vi "DDPoseEst2_AbsTraj_Work.vi"(5 "Track Width FT":dbl, 7 "Max Speed\nFT/SEC":dbl, 8 "Init":bool) -> (0 "AtReference":bool, 1 "Right Speed Target":dbl, 2 "Left Speed Target":dbl, 4 "Odometry Pose Meters":T1={"TRANSLATION"={"X"=0.0, "Y"=0.0}, "ROTATION"={"VALUE"=0.0, "COS"=1.0, "SIN"=0.0}} {"ROTATION"."SIN" format="%13.4f"; "ROTATION"."COS" format="%13.4f"; "ROTATION"."VALUE" format="%13.4f"; "TRANSLATION"."Y" format="%14.3f"; "TRANSLATION"."X" format="%14.3f"})   [LabVIEW 2019]
uses:
  <vilib>/Rock Robotics/WPI/ThirdParty/JAS_Junk/TrajLib/Trajectory_Library.lvlib
  DDPoseEst2_Traj_Globals.vi
  <vilib>/Rock Robotics/WPI/ThirdParty/JAS_Junk/TrajLib/TypeDef/TRANSLATION2D.ctl
  <vilib>/Rock Robotics/WPI/ThirdParty/JAS_Junk/TrajLib/TypeDef/ROTATION2D.ctl
  <vilib>/Rock Robotics/WPI/ThirdParty/JAS_Junk/TrajLib/TypeDef/POSE2D.ctl
  <vilib>/Rock Robotics/WPI/ThirdParty/JAS_Junk/TrajLib/TypeDef/TRAJ_STATE.ctl
  <vilib>/Rock Robotics/WPI/ThirdParty/JAS_Junk/TrajLib/TypeDef/TRAJECTORY.ctl
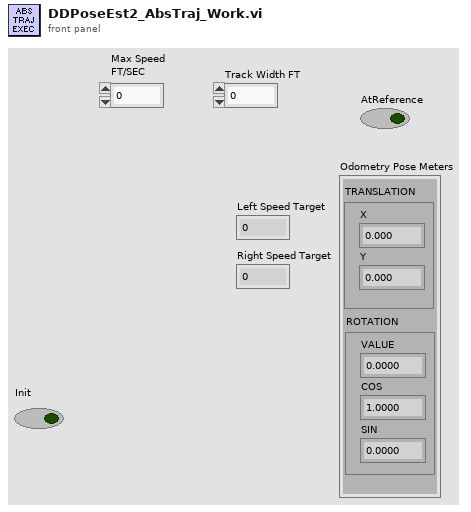
[diagram p1: front panel]
types:
  T1 = typedef "Trajectory_Library.lvlib/POSE2D.ctl" = cluster{"TRANSLATION":T2, "ROTATION":T3}
  T2 = typedef "Trajectory_Library.lvlib/TRANSLATION2D.ctl" = cluster{"X":dbl, "Y":dbl}
  T3 = typedef "Trajectory_Library.lvlib/ROTATION2D.ctl" = cluster{"VALUE":dbl, "COS":dbl, "SIN":dbl}
  T4 = typedef "Trajectory_Library.lvlib/TRAJECTORY.ctl" = cluster{"TotalTImeSecs":dbl, "States":T5[]}
  T5 = typedef "Trajectory_Library.lvlib/TRAJ_STATE.ctl" = cluster{"TimeSeconds":dbl, "Velocity":dbl, "Acceleration":dbl, "POSE":T1, "Curvature":dbl}
  T6 = typedef "Trajectory_Library.lvlib/WEIGHTED_WAYPOINT.ctl" = cluster{"TRANSLATION":T2, "ROTATION":T3, "SCALAR":dbl}
  T7 = typedef "Trajectory_Library.lvlib/RAMSETE_EXE_TUNING.ctl" = cluster{"B":dbl, "Zeta":dbl, "X Tolerance M":dbl, "Y Tolerance M":dbl, "Heading Tolerance RAD":dbl, "Track Width M":dbl, "Max Speed M/S":dbl}
  T8 = typedef "Trajectory_Library.lvlib/RAMSETE.ctl" = cluster{"B":dbl, "Zeta":dbl, "poseTolerance":T1, "poseError":T1, "Enabled":bool}
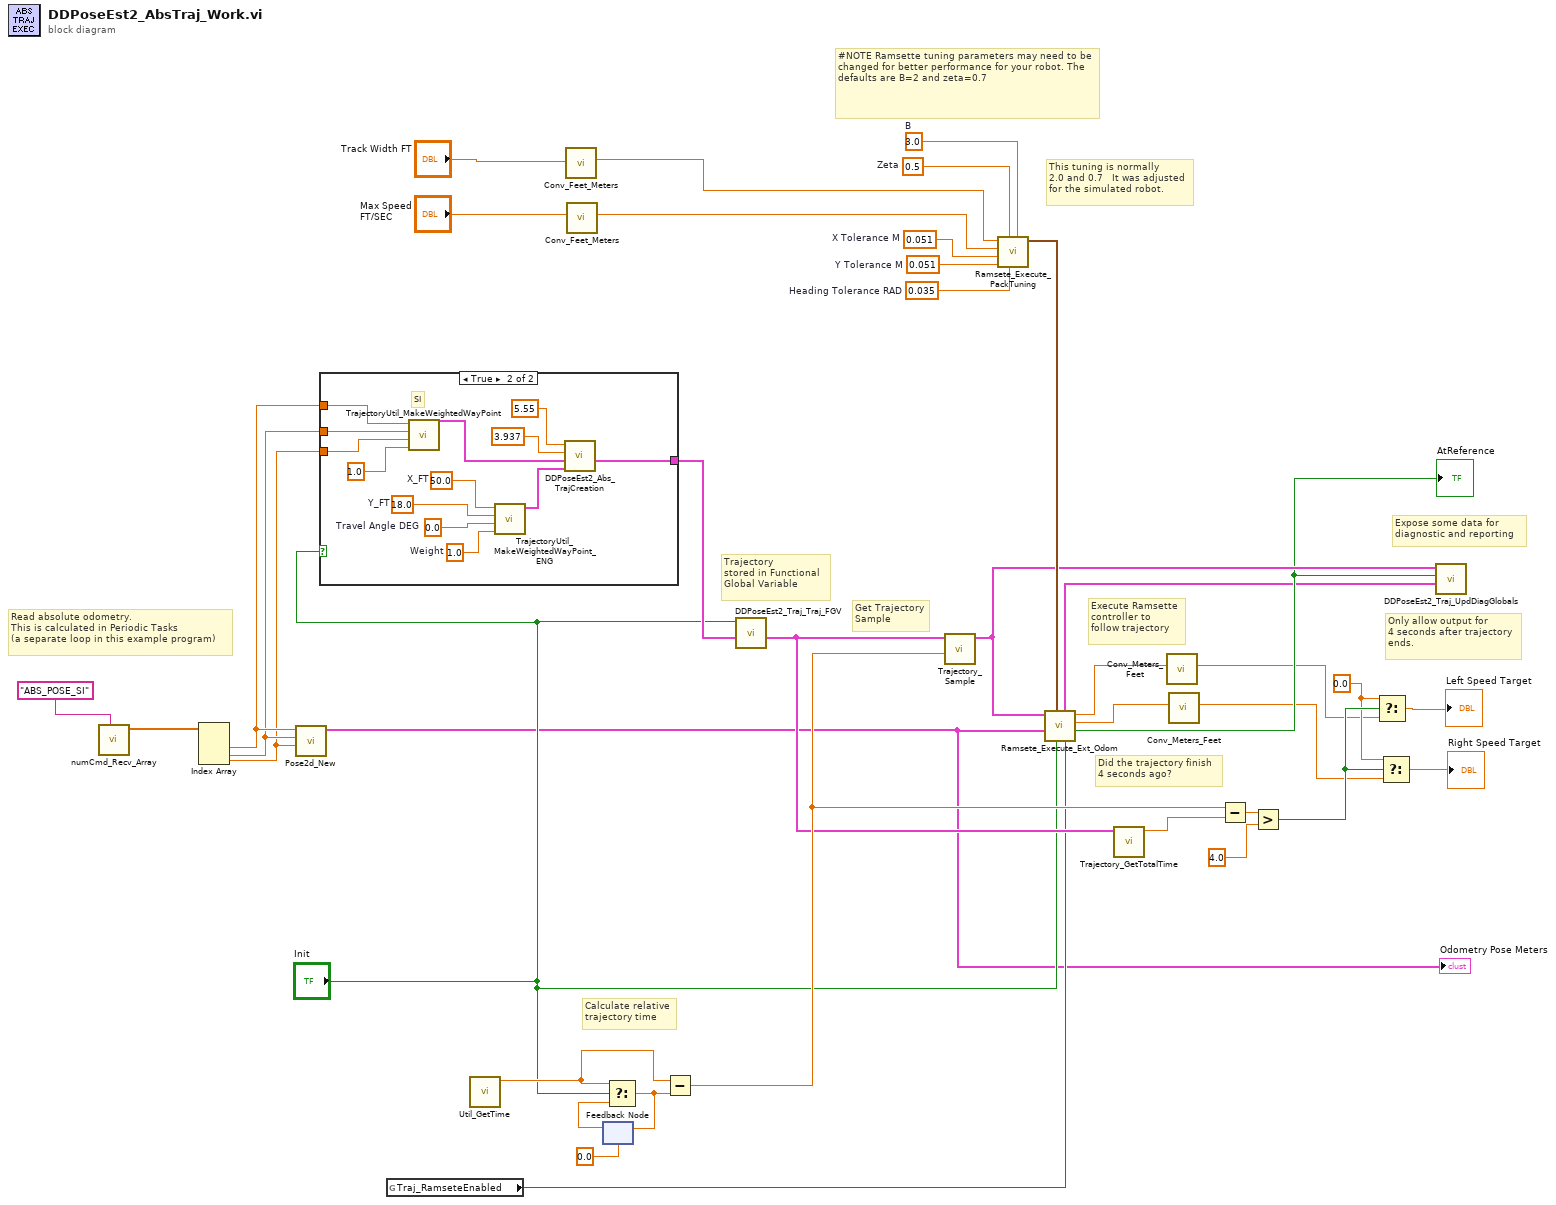
[diagram p0: block diagram]
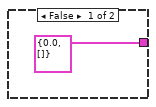
[diagram p2: hidden frame]
diagram:
  w27 = 0.051  # X Tolerance M
  w26 = 0.051  # Y Tolerance M
  w25 = 0.5  # Zeta
  w24 = 0.035  # Heading Tolerance RAD
  w23 = 3.0  # B
  w34 = 0.0 ("t")
  # "Read absolute odometry. \nThis is calculated in Periodic Tasks\n(a separate loop in this example program)"
  # "Execute Ramsette\ncontroller to \nfollow trajectory"
  # "This tuning is normally\n2.0 and 0.7   It was adjusted\nfor the simulated robot."
  # "Expose some data for\ndiagnostic and reporting"
  # "Did the trajectory finish\n4 seconds ago?"
  # "Get Trajectory\nSample"
  # "Trajectory\nstored in Functional\nGlobal Variable"
  # "Calculate relative\ntrajectory time"
  # "#NOTE Ramsette tuning parameters may need to be changed for better performance for your robot. The defaults are B=2 and zeta=0.7"
  # "Only allow output for\n4 seconds after trajectory\nends."
  n1 = call <vilib>:"numCmd_Recv_Array.vi"("Command Name"="ABS_POSE_SI") -> ("Values"=w7:dbl[])  [unwired: 8 in, 2 out]
  n2 = Index Array(array=w7) -> (element #1=w3:dbl, element #2=w2:dbl, element #3=w1:dbl)  [unwired: 3 in]
  n3 = call <vilib>:"Pose2d_New.vi"("Heading"=w1, "Y"=w2, "X"=w3) -> ("out POSe"=w4:T1)  [unwired: 8 in]
  "Odometry Pose Meters" <- w4
  n4 = case shown="True" "Init" {
    tunnel: [T4 {"TotalTImeSecs"=0.0, "States"=[]} ("Absolute Trajectory") w53] -> w6
    tunnel: w3 -> [_ w50]
    tunnel: w2 -> [_ w49]
    tunnel: w1 -> [_ w48]
    frame False {
    }
    frame True {
      w42 = 50.0  # X_FT
      w43 = 18.0  # Y_FT
      w44 = 0.0  # Travel Angle DEG
      w45 = 1.0  # Weight
      # "SI"
      n5 = call <vilib>:"TrajectoryUtil_MakeWeightedWayPoint.vi"("Weight"=1.0, "Travel Angle Radians"=w48, "Y_M"=w49, "X_M"=w50) -> ("WEIGHTED_WAYPOINT"=w46:T6)  [unwired: 7 in]
      n6 = call <vilib>:"TrajectoryUtil_MakeWeightedWayPoint_ENG.vi"("Weight"=w45, "Travel Angle DEG"=w44, "Y_FT"=w43, "X_FT"=w42) -> ("WEIGHTED_WAYPOINT"=w41:T6)  [unwired: 7 in]
      n7 = call "DDPoseEst2_Abs_TrajCreation.vi"("Destination Waypoint"=w41, "Initial Waypoint"=w46, "Effective Track Width Ft"=3.937, "Max Velocity Ft/Sec"=5.55) -> ("Absolute Trajectory"=w53:T4)  [unwired: 4 in, 3 out]
    }
  }
  n8 = global read "DDPoseEst2_Traj_Globals.vi" "Traj_RamseteEnabled"() -> (w18:bool)
  n9 = call <vilib>:"Util_GetTime.vi"() -> ("FPGA_Time_Seconds"=w9:dbl)  [unwired: 9 in, 2 out]
  n10 = call <vilib>:"Conv_Feet_Meters.vi"("Feet"="Track Width FT") -> ("Meters"=w10:dbl)  [unwired: 10 in]
  n11 = call <vilib>:"Conv_Feet_Meters.vi"("Feet"="Max Speed\nFT/SEC") -> ("Meters"=w21:dbl)  [unwired: 10 in]
  n12 = feedback #1(0.0 ("TIME")) -> (w30:dbl)
  n13 = Select(t=w9, s="Init", f=w30) -> (s? t:f=w31:dbl)
  n14 = feedback-in #1(w31) -> ()
  n15 = Subtract(x=w9, y=w31) -> (x-y=w38:dbl)
  n16 = call "DDPoseEst2_Traj_Traj_FGV.vi"("inTRAJECTORY"=w6, "WRITE"="Init") -> ("outTRAJECTORY"=w29:T4)  [unwired: 9 in]
  n17 = call <vilib>:"Trajectory_Sample.vi"("Time"=w38, "InputTRAJECTORY"=w29) -> ("OutputTRAJ_STATE"=w17:T5)  [unwired: 9 in]
  n18 = call <vilib>:"Ramsete_Execute_PackTuning.vi"("B"=w23, "Heading Tolerance RAD"=w24, "Zeta"=w25, "Y Tolerance M"=w26, "X Tolerance M"=w27, "Max Speed M/S"=w21, "Track Width M"=w10) -> ("RAMSETE_EXE_TUNING"=w22:T7)  [unwired: 4 in]
  n19 = call <vilib>:"Ramsete_Execute_Ext_Odom.vi"("Enabled"=w18, "Reset"="Init", "RAMSETE_EXE_TUNING SI"=w22, "Current Pose SI"=w4, "TRAJ_STATE SI"=w17) -> ("AtReference"=w16:bool, "Right Speed Dmd M/S"=w13:dbl, "Left Speed Dmd M/S"=w14:dbl, "outRAMSETE"=w15:T8)  [unwired: 3 in]
  "AtReference" <- w16
  n20 = call <vilib>:"Trajectory_GetTotalTime.vi"("TRAJECTORY"=w29) -> ("TotalTime_Sec"=w28:dbl)  [unwired: 10 in]
  n21 = call <vilib>:"Conv_Meters_Feet.vi"("Meters"=w14) -> ("Feet"=w12:dbl)  [unwired: 10 in]
  n22 = call <vilib>:"Conv_Meters_Feet.vi"("Meters"=w13) -> ("Feet"=w11:dbl)  [unwired: 10 in]
  n23 = Subtract(x=w38, y=w28) -> (x-y=w37:dbl)
  n24 = Greater?(x=w37, y=4.0) -> (0:w35:bool)
  n25 = Select(t=w34, s=w35, f=w12) -> (s? t:f=→"Left Speed Target":dbl)
  n26 = Select(t=w34, s=w35, f=w11) -> (s? t:f=→"Right Speed Target":dbl)
  n27 = call "DDPoseEst2_Traj_UpdDiagGlobals.vi"("outRAMSETE (SI)"=w15, "AtReference"=w16, "OutputTRAJ_STATE (SI)"=w17) -> ()  [unwired: 9 in]
